vi "Reduce.vi"(10 "Failure Descriptions":string[](array[string])) -> (1 "Suffix":string, 2 "Failure Descriptions out":string[](array[string]), 3 "Prefix":string)   [LabVIEW 2017, in "Transparent Assertions.lvlib" / "Constraints.lvlib" / "Binary Operator.lvclass"]
uses:
  Binary Operator.lvclass
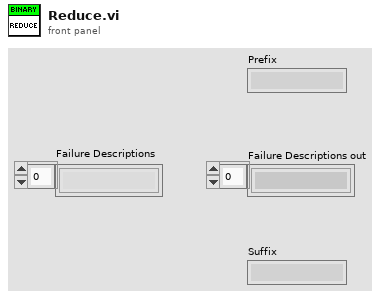
[diagram p1: front panel]
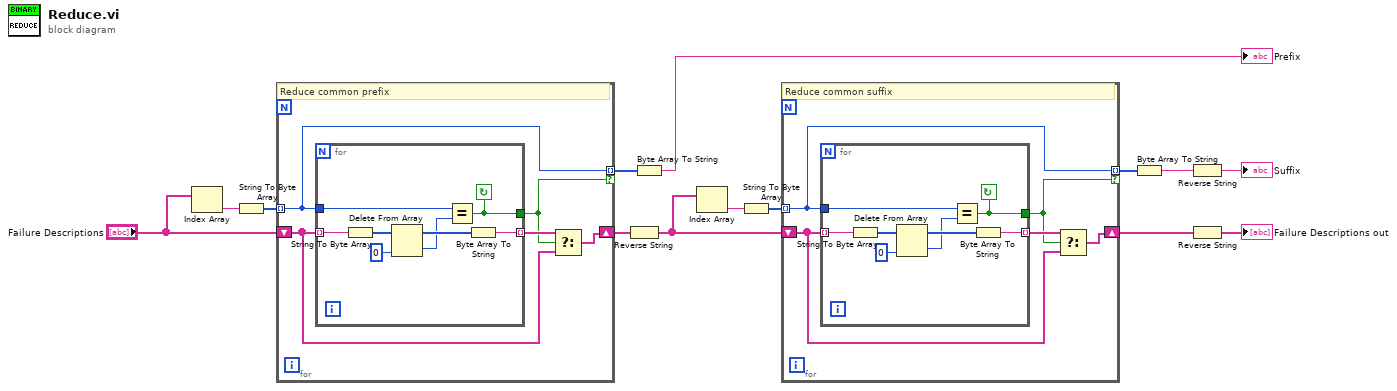
[diagram p0: block diagram]
diagram:
  n1 = Index Array(array="Failure Descriptions") -> (element=w14:string)  [unwired: 1 in]
  n2 = String To Byte Array(string=w14) -> (unsigned byte array=w13:u8[])
  n3 = for {
    tunnel: w13 -> [w15] mode=indexing
    shift-right: [w17] -> w7
    shift-left: "Failure Descriptions" -> [w18]
    tunnel: [w15] -> w11 mode=indexing if=w16
    # "Reduce common prefix"
    n4 = for {
      tunnel: w18 -> [w27] mode=indexing
      tunnel: w15 -> [w25]
      tunnel: [w24] -> w16
      tunnel: [w21] -> w19 mode=indexing
      stop <- w24 continue-if-true
      n5 = String To Byte Array(string=w27) -> (unsigned byte array=w26:u8[])
      n6 = Delete From Array(array=w26, index=0) -> (deleted portion=w20:u8, array with subset deleted=w22:u8[])  [unwired: 1 in]
      n7 = Equal?(x=w25, y=w20) -> (x = y?=w24:bool)
      n8 = Byte Array To String(unsigned byte array=w22) -> (string=w21:string)
    }
    n9 = Select(t=w19, s=w16, f=w18) -> (s? t:f=w17:string[])
  }
  n10 = Reverse String(1:w7) -> (0:w6:string[])
  n11 = Byte Array To String(unsigned byte array=w11) -> (string=→"Prefix":string)
  n12 = Index Array(array=w6) -> (element=w8:string)  [unwired: 1 in]
  n13 = String To Byte Array(string=w8) -> (unsigned byte array=w9:u8[])
  n14 = for {
    tunnel: w9 -> [w28] mode=indexing
    shift-right: [w30] -> w2
    shift-left: w6 -> [w31]
    tunnel: [w28] -> w5 mode=indexing if=w29
    # "Reduce common suffix"
    n15 = for {
      tunnel: w31 -> [w40] mode=indexing
      tunnel: w28 -> [w38]
      tunnel: [w37] -> w29
      tunnel: [w34] -> w32 mode=indexing
      stop <- w37 continue-if-true
      n16 = String To Byte Array(string=w40) -> (unsigned byte array=w39:u8[])
      n17 = Delete From Array(array=w39, index=0) -> (deleted portion=w33:u8, array with subset deleted=w35:u8[])  [unwired: 1 in]
      n18 = Equal?(x=w38, y=w33) -> (x = y?=w37:bool)
      n19 = Byte Array To String(unsigned byte array=w35) -> (string=w34:string)
    }
    n20 = Select(t=w32, s=w29, f=w31) -> (s? t:f=w30:string[])
  }
  n21 = Byte Array To String(unsigned byte array=w5) -> (string=w4:string)
  n22 = Reverse String(1:w4) -> (0:→"Suffix":string)
  n23 = Reverse String(1:w2) -> (0:→"Failure Descriptions out":string[])
